vi "subVI QCam Save File Parameters.vi"(0 "exposure Blue":dbl, 1 "exposure Red":dbl, 2 "exposure":dbl) -> ()   [LabVIEW 2012]
panel:
  out "File String":string
  # "Output"
  # "Input"
  # "Internal Variables"
  # "None"
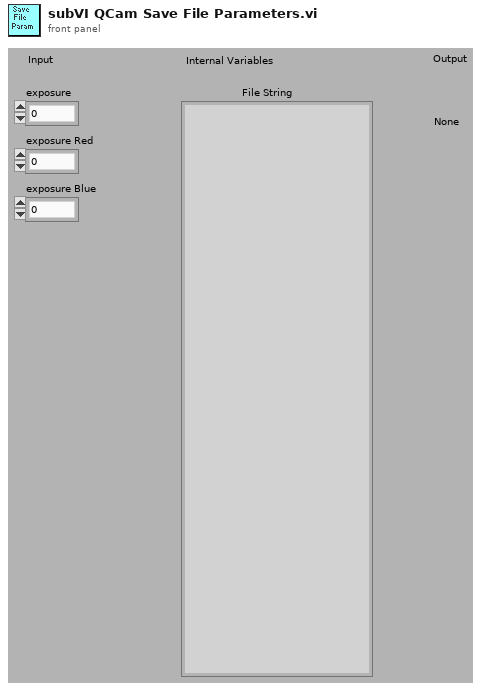
[diagram p1: front panel]
types:
  T1 = enum16{"open", "open or create", "create or replace", "create", "open (read only)"}
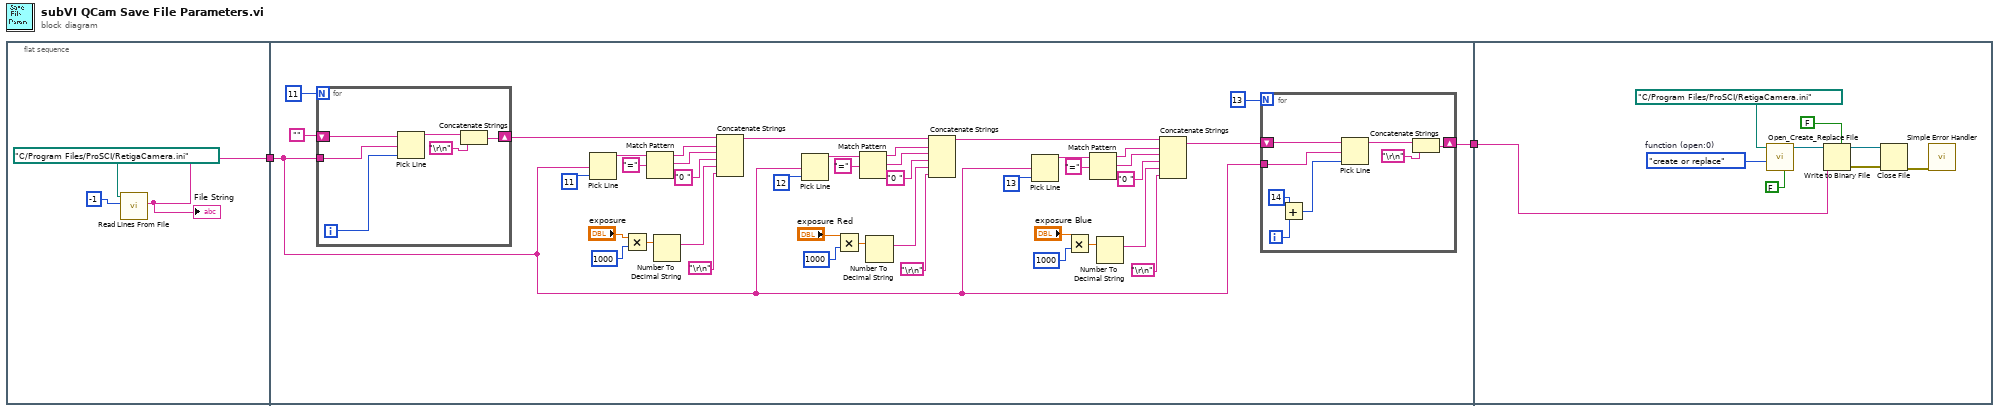
[diagram p0: block diagram]
diagram:
  n1 = flat-sequence {
    tunnel: [w3] -> w2
    tunnel: w2 -> [w7]
    tunnel: [w8] -> w1
    tunnel: w1 -> [w63]
    frame #0 {
      n2 = call <vilib>:"Read Lines From File.vi"("file path (dialog if empty)"=path "C:/Program Files/ProSCI/RetigaCamera.ini", "number of lines (all:-1)"=-1) -> ("line string"=w3:string)  [unwired: 7 out]
      "File String" <- w3
    }
    frame #1 {
      n3 = for {
        N: 11 ("line index") -> [_]
        tunnel: w7 -> [w61]
        shift-right: [w58] -> w39
        shift-left: "" -> [w60]
        i -> [w59]
        n4 = Pick Line(string ("")=w60, multi-line string=w61, line index=w59) -> (output string=w57:string)
        n5 = Concatenate Strings(w57, "\r\n") -> (w58:string)
      }
      n6 = Pick Line(multi-line string=w7, line index=11) -> (output string=w44:string)  [unwired: 1 out]
      n7 = Multiply(x="exposure", y=1000) -> (x*y=w40:dbl)
      n8 = Match Pattern(string=w44, regular expression="=") -> (before substring=w38:string, match substring=w37:string)  [unwired: 3 out]
      n9 = Number To Decimal String(number=w40) -> (decimal integer string=w35:string)  [unwired: 1 out]
      n10 = Concatenate Strings(w39, w38, w37, "0 " ("string"), w35, "\r\n") -> (w22:string)
      n11 = Pick Line(multi-line string=w7, line index=12) -> (output string=w32:string)  [unwired: 1 out]
      n12 = Multiply(x="exposure Red", y=1000) -> (x*y=w29:dbl)
      n13 = Match Pattern(string=w32, regular expression="=") -> (before substring=w28:string, match substring=w27:string)  [unwired: 3 out]
      n14 = Number To Decimal String(number=w29) -> (decimal integer string=w25:string)  [unwired: 1 out]
      n15 = Concatenate Strings(w22, w28, w27, "0 " ("string"), w25, "\r\n") -> (w11:string)
      n16 = Pick Line(multi-line string=w7, line index=13) -> (output string=w21:string)  [unwired: 1 out]
      n17 = Multiply(x="exposure Blue", y=1000) -> (x*y=w18:dbl)
      n18 = Match Pattern(string=w21, regular expression="=") -> (before substring=w17:string, match substring=w16:string)  [unwired: 3 out]
      n19 = Number To Decimal String(number=w18) -> (decimal integer string=w14:string)  [unwired: 1 out]
      n20 = Concatenate Strings(w11, w17, w16, "0 " ("string"), w14, "\r\n") -> (w9:string)
      n21 = for {
        N: 13 ("line index") -> [_]
        tunnel: w7 -> [w55]
        shift-right: [w48] -> w8
        shift-left: w9 -> [w54]
        i -> [w53]
        n22 = Add(x=14, y=w53) -> (x+y=w51:i32)
        n23 = Pick Line(string ("")=w54, multi-line string=w55, line index=w51) -> (output string=w49:string)
        n24 = Concatenate Strings(w49, "\r\n") -> (w48:string)
      }
    }
    frame #2 {
      w69 = T1."create or replace"  # function (open:0)
      n25 = call <vilib>:"Open_Create_Replace File.vi"("advisory dialog? (display:T)"=FALSE, "function (open:0)"=w69, "file path"=path "C:/Program Files/ProSCI/RetigaCamera.ini") -> ("refnum"=w68:refnum<file>)  [unwired: 4 in, 4 out]
      n26 = Write to Binary File(file (use dialog)=w68, data=w63, 5:FALSE ("prepend array or string size? (T)")) -> (refnum out=w67:refnum<file>, error out=w66:errorcluster)  [unwired: 1 in, 3 out]
      n27 = Close File(refnum=w67, error in=w66) -> (error out=w65:errorcluster)  [unwired: 1 out]
      n28 = call <vilib>:"Simple Error Handler.vi"("error in (no error)"=w65) -> ()  [unwired: 1 in, 8 out]
    }
  }
